vi "Autonomous Independent.vi"() -> ()   [LabVIEW 2014]
doc: "This VI is called when autonomous begins, and will automatically be terminated when autonomous ends. You can carry out timed or sensor driven robot movement independently without needing to return to the caller."
uses:
  <vilib>/Rock Robotics/WPI/DriverStation/WPI_DriverStationDerivedRobotMode.ctl
  <vilib>/Rock Robotics/WPI/DriverStation/WPI_DriverStationMatch Info.ctl
  Global Variables.vi
  <vilib>/Utility/file.llb/Read From Spreadsheet File (DBL).vi
  <vilib>/addons/control/pid/pid.llb/PID (DBL).vi
  <vilib>/Utility/file.llb/Write To Spreadsheet File (DBL).vi
  <vilib>/addons/control/pid/NI_PID_pid.lvlib
panel:
  in  "output range":cluster{"output high":dbl, "output low":dbl}={"output high"=1.5, "output low"=0.5} {"output low" format="%.2f"; "output high" format="%.2f"}
  in  "PID gains":T1={"proportional gain (Kc)"=1.0, "integral time (Ti, min)"=0.01, "derivative time (Td, min)"=0.0} {"derivative time (Td, min)" format="%.3f"; "integral time (Ti, min)" format="%.3f"; "proportional gain (Kc)" format="%.3f"}
  in  "Match Info":T2={"Autonomous Elapsed Seconds"=0.0, "TeleOp Elapsed Seconds"=0.0, "Disabled Elapsed Seconds"=0.0, "Visited Autonomous"=FALSE, "Visited TeleOp"=FALSE, "Visited Disabled"=FALSE, "Autonomous Settings"={"Autonomous Style"=enum."Independent", "VI Refnum"=refnum}}
  in  "Call Context":T3
  # "Be sure to right-click and choose Data Operations>>Make Current Value default if you want to save the array values with the VI"
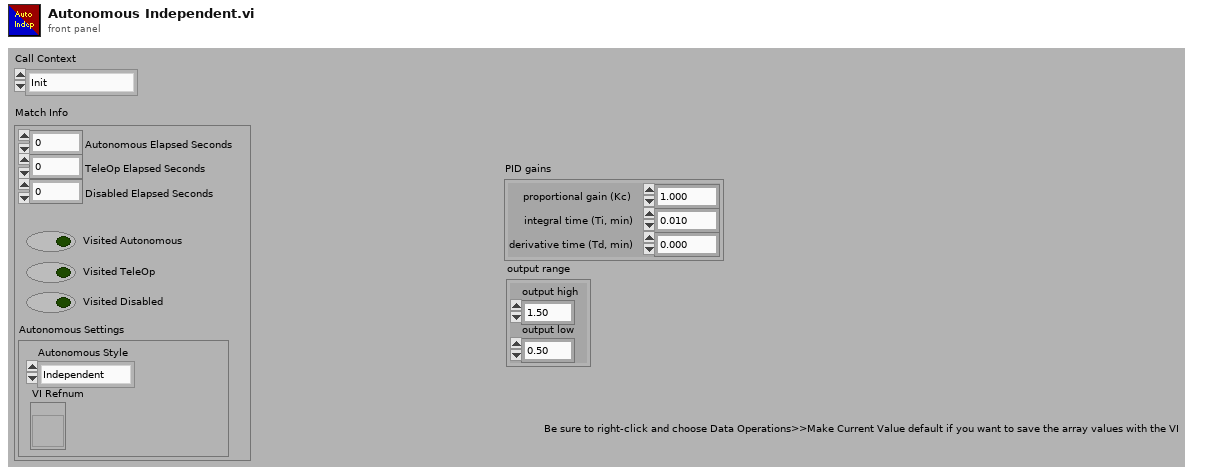
[diagram p1: front panel]
types:
  T1 = cluster{"proportional gain (Kc)":dbl, "integral time (Ti, min)":dbl, "derivative time (Td, min)":dbl}
  T2 = typedef "WPI_DriverStationMatch Info.ctl" = cluster{"Autonomous Elapsed Seconds":dbl, "TeleOp Elapsed Seconds":dbl, "Disabled Elapsed Seconds":dbl, "Visited Autonomous":bool, "Visited TeleOp":bool, "Visited Disabled":bool, "Autonomous Settings":cluster{"Autonomous Style":enum16{"Iterative", "Independent"}, "VI Refnum":refnum<vi>}}
  T3 = typedef "WPI_DriverStationDerivedRobotMode.ctl" = enum16{"Init", "Execute", "Stop"}
  T4 = typedef "WPI_JoystickDevRef.ctl" = cluster{"Device":T5}
  T5 = typedef "WPI_JoystickDeviceEnum.ctl" = enum16{"USB 0", "USB 1", "USB 2", "USB 3", "USB 4", "USB 5"}
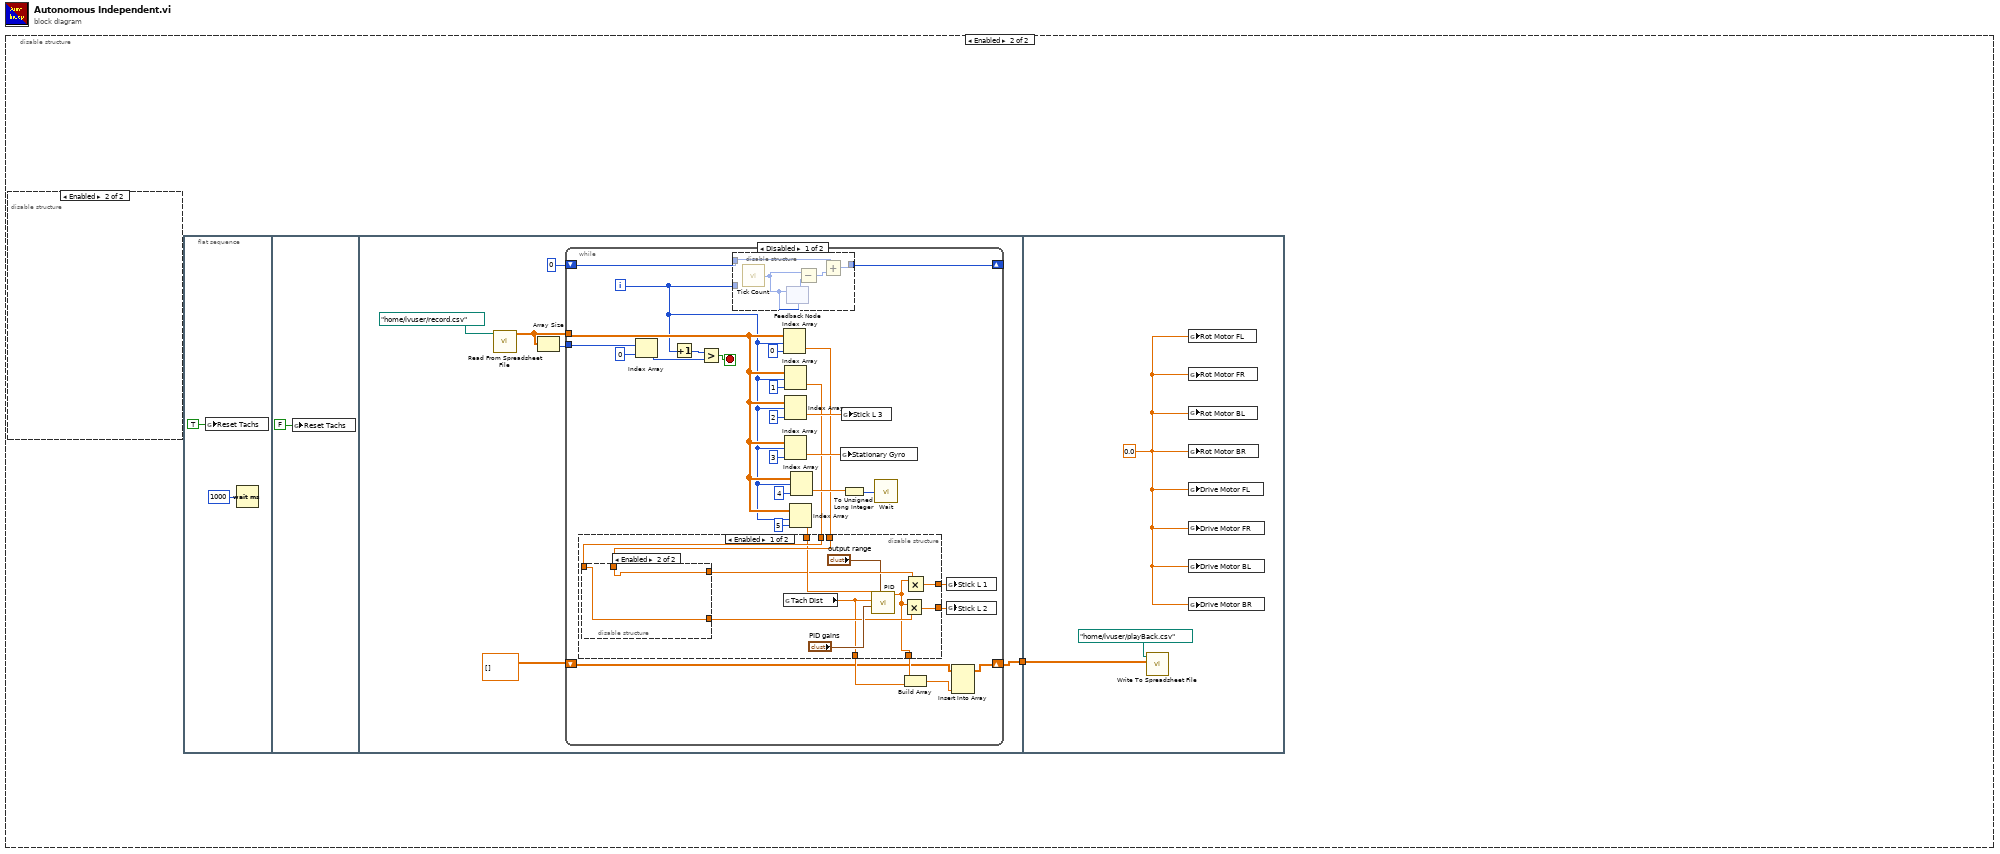
[diagram p0: block diagram]
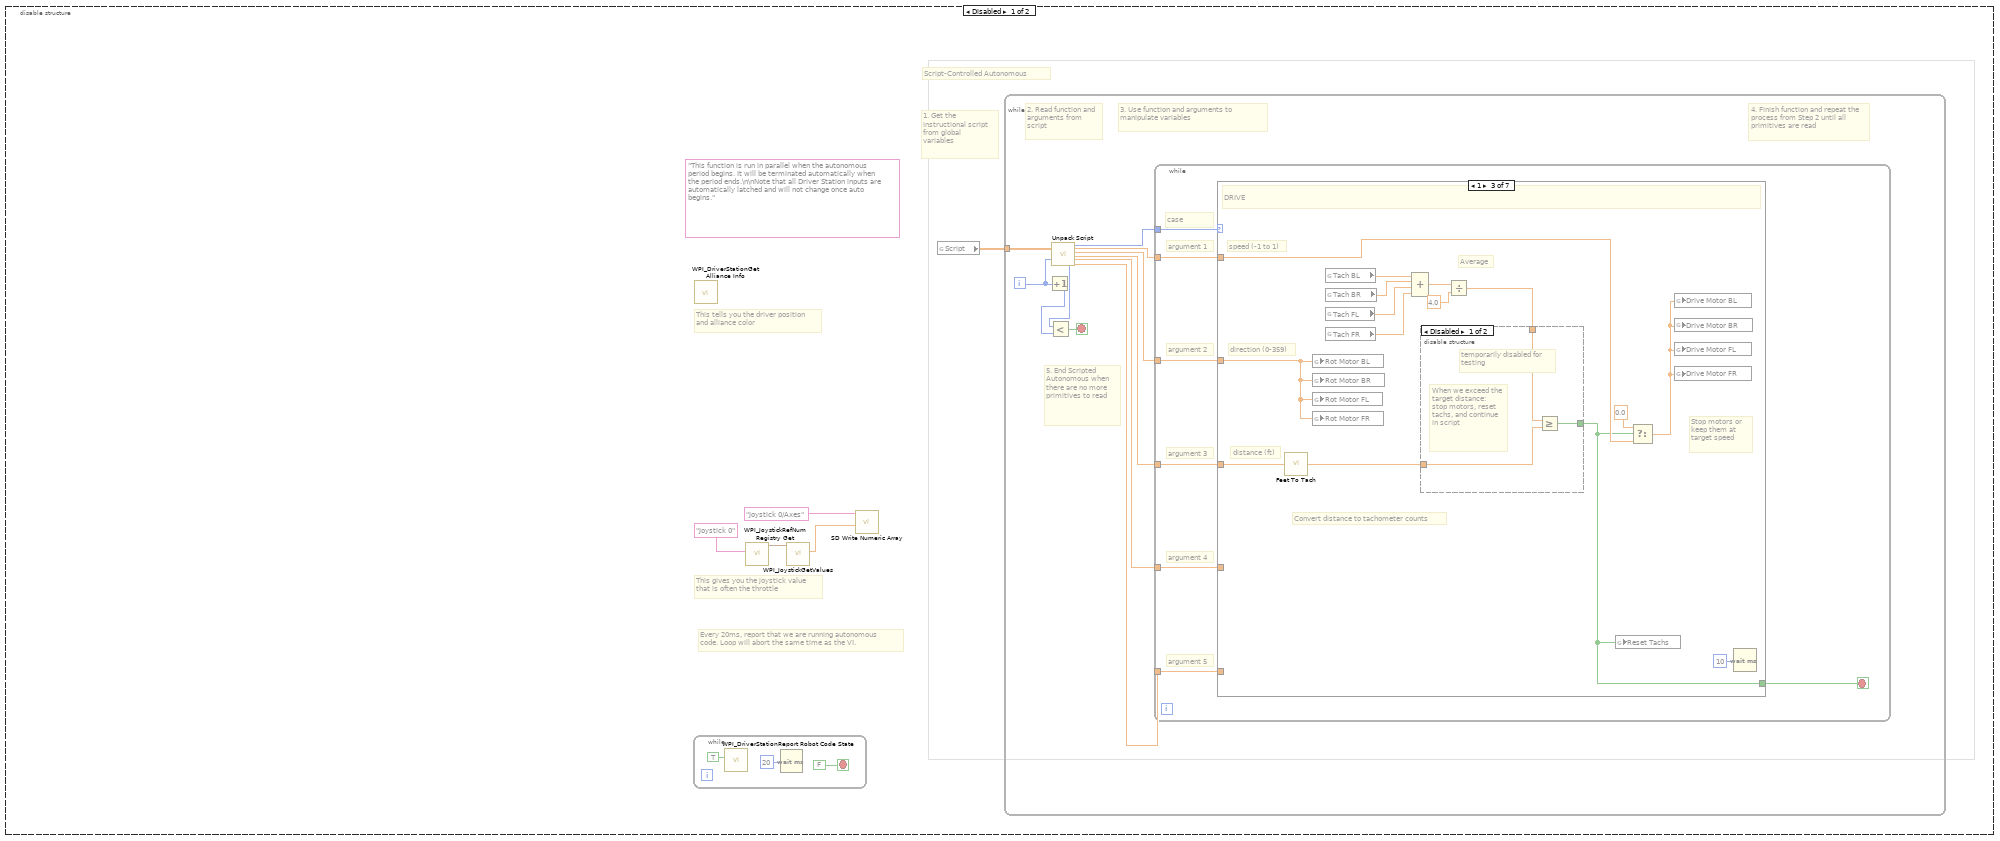
[diagram p2: hidden frame]
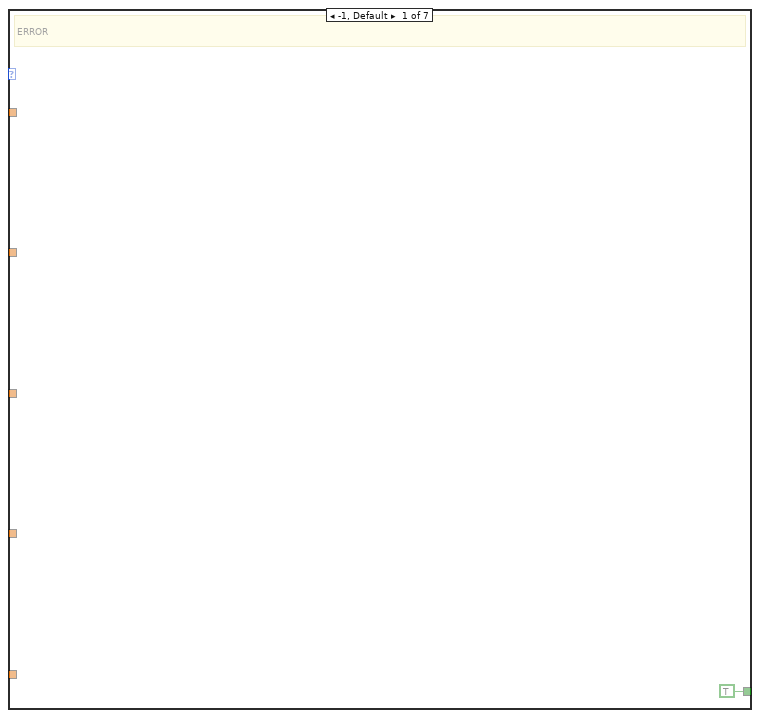
[diagram p3: hidden frame]
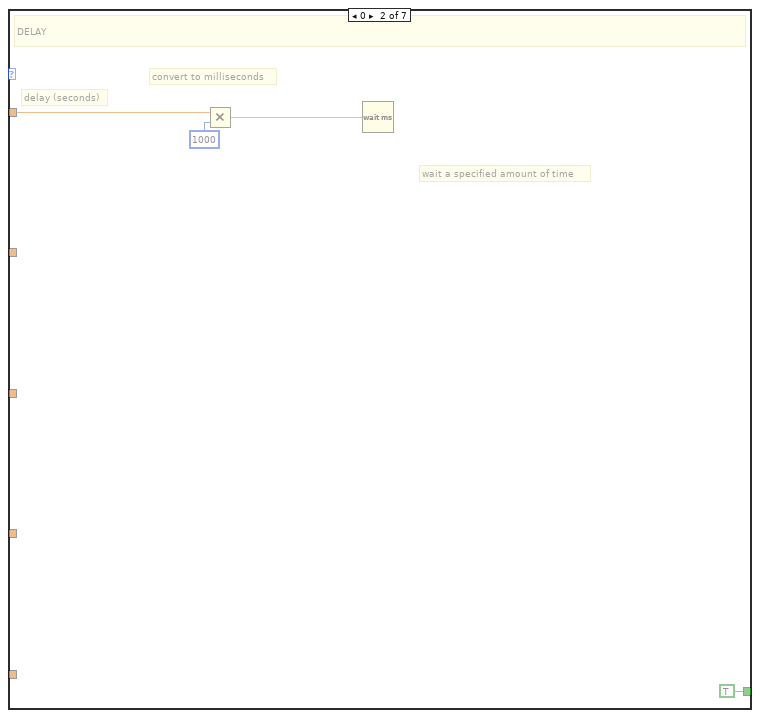
[diagram p4: hidden frame]
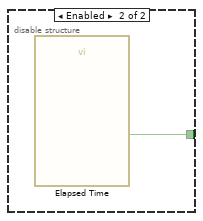
[diagram p5: hidden frame]
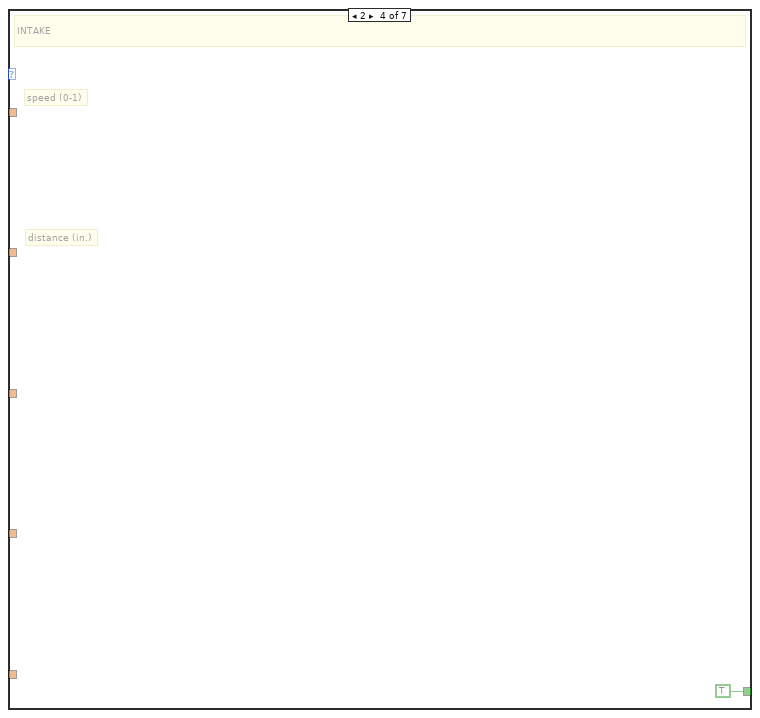
[diagram p6: hidden frame]
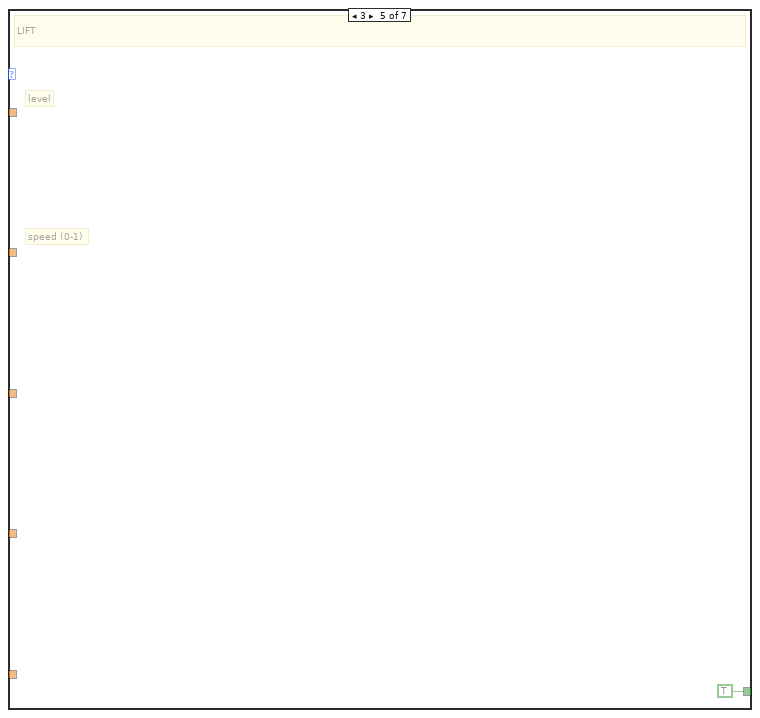
[diagram p7: hidden frame]
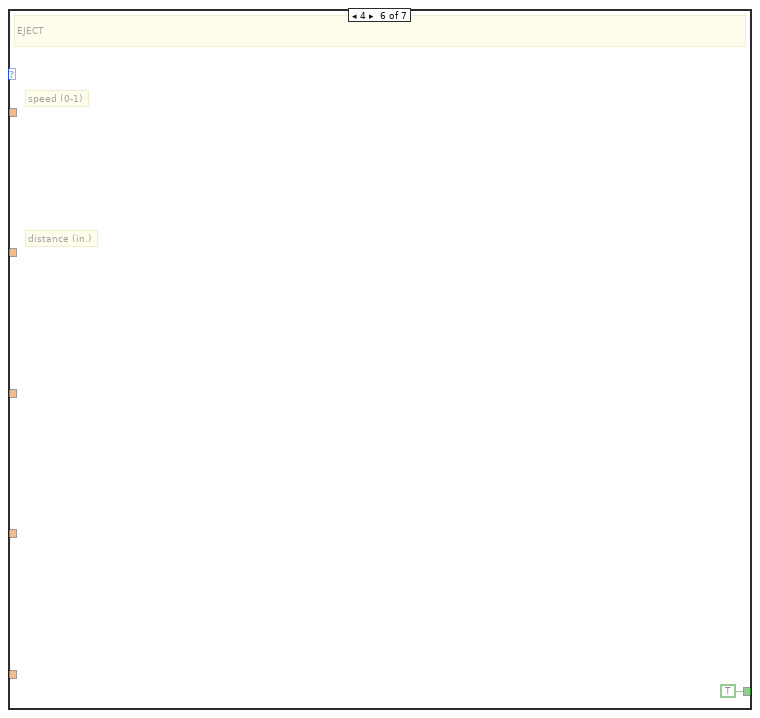
[diagram p8: hidden frame]
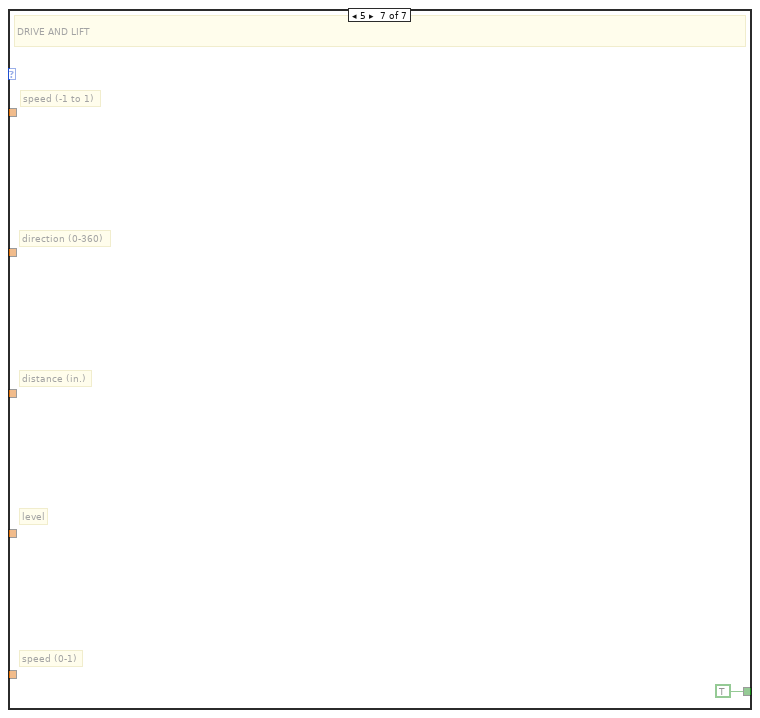
[diagram p9: hidden frame]
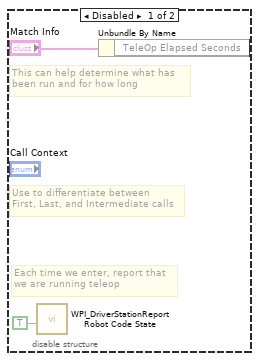
[diagram p10: hidden frame]
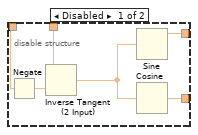
[diagram p11: hidden frame]
diagram:
  n1 = disable-structure shown="Enabled" {
    frame Disabled {
      (unwired) "This function is run in parallel when the autonomous period begins. It will be terminated automatically when the period ends.\n\nNote that all Driver Station inputs are automatically latched and will not change once auto begins."
      # "1. Get the instructional script from global variables"
      # "Script-Controlled Autonomous"
      # "Every 20ms, report that we are running autonomous\ncode. Loop will abort the same time as the VI."
      # "This gives you the joystick value\nthat is often the throttle"
      # "This tells you the driver position\nand alliance color"
      n2 = while {
        stop <- FALSE stop-if-true
        n3 = call <vilib>:"WPI_DriverStationReport Robot Code State.vi"("Autonomous"=TRUE) -> ()  [unwired: 10 in, 1 out]
        n4 = Wait (ms)(milliseconds to wait=u32 20) -> ()  [unwired: 1 out]
      }
      n5 = call <vilib>:"WPI_DriverStationGet Alliance Info.vi"() -> ()  [unwired: 12 out]
      n6 = call <vilib>:"WPI_JoystickRefNum Registry Get.vi"("refnum name"="Joystick 0") -> ("JoystickDevRef"=w4:T4)  [unwired: 1 in, 9 out]
      n7 = call <vilib>:"WPI_JoystickGetValues.vi"("JoystickDevRef"=w4) -> ("Axes"=w2:dbl[])  [unwired: 6 in, 4 out]
      n8 = call <vilib>:"SD Write Numeric Array.vi"("Numeric Array"=w2, "Name"="Joystick 0/Axes") -> ()  [unwired: 8 in, 2 out]
      n9 = global read "Global Variables.vi" "Script"() -> (w1:dbl[][])
      n10 = while {
        tunnel: w1 -> [w6]
        i -> [w10]
        stop <- w16 stop-if-true
        # "4. Finish function and repeat the process from Step 2 until all primitives are read"
        # "3. Use function and arguments to manipulate variables"
        # "5. End Scripted Autonomous when there are no more primitives to read"
        # "2. Read function and arguments from script"
        n11 = Increment(x=w10) -> (x+1=w8:i32)
        n12 = call "Unpack Script.vi"("script"=w6, "index"=w10) -> ("# of primitives"=w7:i32, "primitive"=w9:i32, "argument 1"=w15:dbl, "argument 2"=w14:dbl, "argument 3"=w13:dbl, "argument 4"=w12:dbl, "argument 5"=w11:dbl)  [unwired: 11 in]
        n13 = Less?(x=w7, y=w8) -> (x < y?=w16:bool)
        n14 = while {
          tunnel: w15 -> [w23]
          tunnel: w14 -> [w22]
          tunnel: w13 -> [w21]
          tunnel: w12 -> [w20]
          tunnel: w11 -> [w19]
          tunnel: w9 -> [w18]
          stop <- w17 stop-if-true
          # "case"
          # "argument 5"
          # "argument 4"
          # "argument 3"
          # "argument 2"
          # "argument 1"
          n15 = case shown="1" w18 {
            tunnel: w23 -> [_ w27 w34 _ _ _ _]
            tunnel: w22 -> [_ _ w31 _ _ _ _]
            tunnel: w21 -> [_ _ w43 _ _ _ _]
            tunnel: w20 -> [_ _ _ _ _ _ _]
            tunnel: w19 -> [_ _ _ _ _ _ _]
            tunnel: [TRUE TRUE w29 TRUE TRUE TRUE TRUE] -> w17
            frame -1, Default {
              # "ERROR"
            }
            frame 0 {
              # "wait a specified amount of time"
              # "convert to milliseconds"
              # "delay (seconds)"
              # "DELAY"
              n16 = Multiply(x=w27, y=1000) -> (x*y=w26:dbl)
              n17 = Wait (ms)(milliseconds to wait=w26) -> ()  [unwired: 1 out]
            }
            frame 1 {
              # "Stop motors or keep them at target speed"
              # "Average"
              # "Convert distance to tachometer counts"
              # "distance (ft)"
              # "direction (0-359)"
              # "speed (-1 to 1)"
              # "DRIVE"
              n18 = call "Feet To Tach.vi"("Feet"=w43) -> ("Tach Counts"=w35:dbl)
              n19 = global write "Global Variables.vi" "Rot Motor BL"(w31) -> ()
              n20 = global write "Global Variables.vi" "Rot Motor BR"(w31) -> ()
              n21 = global write "Global Variables.vi" "Rot Motor FL"(w31) -> ()
              n22 = global write "Global Variables.vi" "Rot Motor FR"(w31) -> ()
              n23 = global read "Global Variables.vi" "Tach BL"() -> (w42:dbl)
              n24 = global read "Global Variables.vi" "Tach BR"() -> (w41:dbl)
              n25 = global read "Global Variables.vi" "Tach FL"() -> (w40:dbl)
              n26 = global read "Global Variables.vi" "Tach FR"() -> (w39:dbl)
              n27 = Compound Arithmetic op=ADD(w42, w41, w40, w39) -> (w38:dbl)
              n28 = Divide(x=w38, y=4.0) -> (x/y=w36:dbl)
              n29 = disable-structure shown="Disabled" {
                disable-tunnel: w36 -> [w46 _]
                disable-tunnel: w35 -> [w45 _]
                disable-tunnel: [w44 w47] -> w29
                frame Disabled {
                  # "When we exceed the target distance: stop motors, reset tachs, and continue in script"
                  # "temporarily disabled for\ntesting"
                  n30 = Greater Or Equal?(x=w46, y=w45) -> (x >= y?=w44:bool)
                }
                frame Enabled {
                  n31 = call "Elapsed Time"() -> ("Time has Elapsed"=w47:bool)  [unwired: 12 in, 7 out]
                }
              }
              n32 = global write "Global Variables.vi" "Reset Tachs"(w29) -> ()
              n33 = Select(t=0.0, s=w29, f=w34) -> (s? t:f=w32:dbl)
              n34 = global write "Global Variables.vi" "Drive Motor BL"(w32) -> ()
              n35 = global write "Global Variables.vi" "Drive Motor BR"(w32) -> ()
              n36 = global write "Global Variables.vi" "Drive Motor FL"(w32) -> ()
              n37 = global write "Global Variables.vi" "Drive Motor FR"(w32) -> ()
              n38 = Wait (ms)(milliseconds to wait=u32 10) -> ()  [unwired: 1 out]
            }
            frame 2 {
              # "distance (in.)"
              # "speed (0-1)"
              # "INTAKE"
            }
            frame 3 {
              # "speed (0-1)"
              # "level"
              # "LIFT"
            }
            frame 4 {
              # "distance (in.)"
              # "speed (0-1)"
              # "EJECT"
            }
            frame 5 {
              # "speed (0-1)"
              # "level"
              # "distance (in.)"
              # "direction (0-360)"
              # "speed (-1 to 1)"
              # "DRIVE AND LIFT"
            }
          }
        }
      }
    }
    frame Enabled {
      n39 = disable-structure shown="Enabled" {
        frame Disabled {
          # "Each time we enter, report that\nwe are running teleop"
          # "Use to differentiate between\nFirst, Last, and Intermediate calls"
          # "This can help determine what has\nbeen run and for how long"
          n40 = call <vilib>:"WPI_DriverStationReport Robot Code State.vi"("TeleOp"=TRUE ("Autonomous")) -> ()  [unwired: 10 in, 1 out]
          n41 = Unbundle By Name("Match Info") -> ()  [unwired: 1 out]
        }
        frame Enabled {
        }
      }
      n42 = flat-sequence {
        tunnel: [w61] -> w55
        tunnel: w55 -> [w124]
        frame #0 {
          n43 = global write "Global Variables.vi" "Reset Tachs"(TRUE ("Reset Tachs")) -> ()
          n44 = Wait (ms)(milliseconds to wait=u32 1000) -> ()  [unwired: 1 out]
        }
        frame #1 {
          n45 = global write "Global Variables.vi" "Reset Tachs"(FALSE ("Reset Tachs")) -> ()
        }
        frame #2 {
          n46 = call-poly <vilib>:"Read From Spreadsheet File.vi"("file path (dialog if empty)"=path "/home/lvuser/record.csv") -> ("all rows"=w65:dbl[][])  [unwired: 6 in, 4 out]
          n47 = Array Size(array=w65) -> (size(s)=w66:i32[])
          n48 = while {
            tunnel: w65 -> [w78]
            tunnel: w66 -> [w91]
            shift-right: [w77] -> _
            shift-left: u32 0 -> [w88]
            shift-right: [w68] -> w61
            shift-left: dbl[][] [] -> [w67]
            i -> [w72]
            stop <- w86 stop-if-true
            n49 = Index Array(array=w91, index=0) -> (element=w89:i32)
            n50 = Increment(x=w72) -> (x+1=w92:i32)
            n51 = Greater?(x=w92, y=w89) -> (0:w86:bool)
            n52 = disable-structure shown="Disabled" {
              disable-tunnel: w88 -> [w118 w122]
              disable-tunnel: [w117 w122] -> w77
              disable-tunnel: w72 -> [_ _]
              frame Disabled {
                n53 = call "Tick Count"() -> ("Tick Count(mSec)"=w120:u32)
                n54 = feedback #1(w120) -> (w121:u32)
                n55 = feedback-in #1(w120) -> ()
                n56 = Subtract(x=w120, y=w121) -> (x-y=w119:u32)
                n57 = Add(x=w118, y=w119) -> (x+y=w117:u32)
              }
              frame Enabled {
              }
            }
            n58 = Index Array(array=w78, index (row)=w72, index (col)=0 ("disabled index (col)")) -> (element=w80:dbl)
            n59 = Index Array(array=w78, index (row)=w72, index (col)=1) -> (element=w79:dbl)
            n60 = Index Array(array=w78, index (row)=w72, index (col)=2) -> (element=w87:dbl)
            n61 = Index Array(array=w78, index (row)=w72, index (col)=3) -> (element=w84:dbl)
            n62 = Index Array(array=w78, index (row)=w72, index (col)=5 ("disabled index (col)")) -> (element=w75:dbl)
            n63 = disable-structure shown="Enabled" {
              disable-tunnel: w80 -> [w106 w116]
              disable-tunnel: w79 -> [w105 w115]
              disable-tunnel: w75 -> [w103 _]
              disable-tunnel: [w101 w116] -> w74
              disable-tunnel: [w99 w115] -> w73
              disable-tunnel: [w97 _] -> w71
              disable-tunnel: [w96 _] -> w70
              frame Enabled {
                n64 = disable-structure shown="Enabled" {
                  disable-tunnel: w106 -> [w112 w113]
                  disable-tunnel: w105 -> [w110 w114]
                  disable-tunnel: [w108 w114] -> w98
                  disable-tunnel: [w107 w113] -> w102
                  frame Disabled {
                    n65 = Negate(x=w110) -> (-x=w111:dbl)
                    n66 = Inverse Tangent (2 Input)(1:w111, 2:w112) -> (0:w109:dbl)
                    n67 = Sine(x=w109) -> (sin(x)=w107:dbl)
                    n68 = Cosine(x=w109) -> (cos(x)=w108:dbl)
                  }
                  frame Enabled {
                  }
                }
                n69 = global read "Global Variables.vi" "Tach Dist"() -> (w96:dbl)
                n70 = call-poly <vilib>:"PID.vi"("output range"="output range", "PID gains"="PID gains", "process variable"=w96, "setpoint"=w103) -> ("output"=w97:dbl)  [unwired: 6 in, 1 out]
                n71 = Multiply(x=w97, y=w98) -> (x*y=w99:dbl)
                n72 = Multiply(x=w97, y=w102) -> (x*y=w101:dbl)
              }
              frame Disabled {
              }
            }
            n73 = Index Array(array=w78, index (row)=w72, index (col)=4) -> (element=w82:dbl)
            n74 = global write "Global Variables.vi" "Stationary Gyro"(w84) -> ()
            n75 = global write "Global Variables.vi" "Stick L 3"(w87) -> ()
            n76 = To Unsigned Long Integer(number=w82) -> (unsigned 32bit integer=w81:u32)
            n77 = call "Wait"("Count(mSec)"=w81) -> ()  [unwired: 1 out]
            n78 = Build Array(w71, w70) -> (w69:dbl[])
            n79 = global write "Global Variables.vi" "Stick L 1"(w74) -> ()
            n80 = global write "Global Variables.vi" "Stick L 2"(w73) -> ()
            n81 = Insert Into Array(array=w67, new element=w69) -> (w68:dbl[][])  [unwired: 2 in]
          }
        }
        frame #3 {
          w125 = 0.0
          n82 = call-poly <vilib>:"Write To Spreadsheet File.vi"("2D data"=w124, "file path (dialog if empty)"=path "/home/lvuser/playBack.csv") -> ()  [unwired: 6 in, 1 out]
          n83 = global write "Global Variables.vi" "Rot Motor FL"(w125) -> ()
          n84 = global write "Global Variables.vi" "Rot Motor FR"(w125) -> ()
          n85 = global write "Global Variables.vi" "Rot Motor BL"(w125) -> ()
          n86 = global write "Global Variables.vi" "Rot Motor BR"(w125) -> ()
          n87 = global write "Global Variables.vi" "Drive Motor FL"(w125) -> ()
          n88 = global write "Global Variables.vi" "Drive Motor FR"(w125) -> ()
          n89 = global write "Global Variables.vi" "Drive Motor BL"(w125) -> ()
          n90 = global write "Global Variables.vi" "Drive Motor BR"(w125) -> ()
        }
      }
    }
  }
